vi "Init Msg.vi"(10 "Msg Input":refnum<class "Msg Input.lvclass">) -> (2 "Msg":refnum<class "Msg.lvclass">)   [LabVIEW 2025, in "_Template.lvlib" / "Templates.lvlib" / "TEMPLATE Msg.lvlib" / "TEMPLATE Msg.lvlib"]
uses:
  TEMPLATE Msg.lvlib
  jettl/jettl/Msg/Msg.lvclass
  jettl/jettl/Msg Input/Msg Input.lvclass
  TEMPLATE Msg/TEMPLATE Msg.lvclass
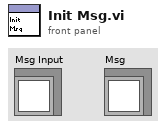
[diagram p1: front panel]
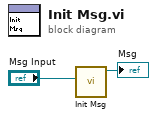
[diagram p0: block diagram]
diagram:
  n1 = call "Init Msg.vi"("Msg Input"="Msg Input") -> ("TEMPLATE Msg out"=→"Msg":refnum<class "TEMPLATE Msg.lvclass">)  [unwired: 10 in]
